vi "STM Set Meta Data (Serial Ref).vi"(7 "Meta data":T1[](array[typedef]), 8 "error in":errorcluster, 11 "VISA resource name":refnum<visa-resource-name>) -> (0 "error out":errorcluster, 3 "Connection Info Out":T2)   [LabVIEW 2010]
doc: "Assigns the meta data cluster associated with this STM session.\n\nCopyright 2015, 2016, 2017 National Instruments Corporation\n\nLicensed under the Apache License, Version 2.0 (the \"License\"); you may not use this file except in compliance with the License.\n\n You may obtain a copy of the License at\n\n http://www.apache.org/licenses/LICENSE-2.0\n\nUnless required by applicable law or agreed to in writing, software distributed under the License is distributed on an \"AS IS\" BASIS, WITHOUT WARRANTIES OR CONDITIONS OF ANY KIND, either express or implied.\n\nSee the License for the specific language governing permissions and limitations under the License."
uses:
  stm_Serial Connection Info.ctl
  stm_MetaDataElement.ctl
  NI STM.lvlib
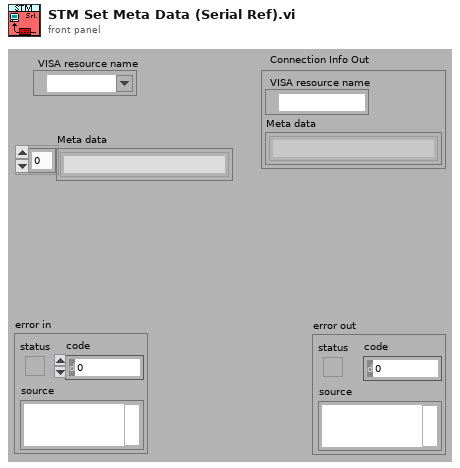
[diagram p1: front panel]
types:
  T1 = typedef "stm_MetaDataElement.ctl" = string
  T2 = typedef "stm_Serial Connection Info.ctl" = cluster{"VISA resource name":refnum<visa-resource-name>, "Meta data":T1[]}
  T3 = typedef "NI STM.lvlib/Serial Connection Info.ctl" = cluster{"VISA resource name":refnum<visa-resource-name>, "meta data":T4[]}
  T4 = typedef "NI STM.lvlib/MetaDataElement.ctl" = string
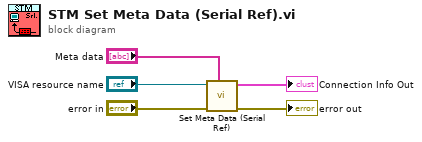
[diagram p0: block diagram]
diagram:
  n1 = call "Set Meta Data (Serial Ref).vi"("meta data"="Meta data", "error in"="error in", "VISA resource name"="VISA resource name") -> ("error out"=→"error out":errorcluster, "connection info out"=→"Connection Info Out":T3)  [unwired: 7 in]
